vi "process_maxes.vi"(1 "Parsed formula node reference fn 2nd derivative":T1 {"Y Values" format="%.2f"}, 2 "Maxes":dbl[][](array[numeric]), 3 "Wavelengths":dbl[](array[numeric])) -> (0 "Phase''":dbl[](array[numeric]))   [LabVIEW 2022 SP3]
uses:
  <vilib>/gmath/NI_Gmath.lvlib
panel:
  # "operator"
  # "register1"
  # "register2"
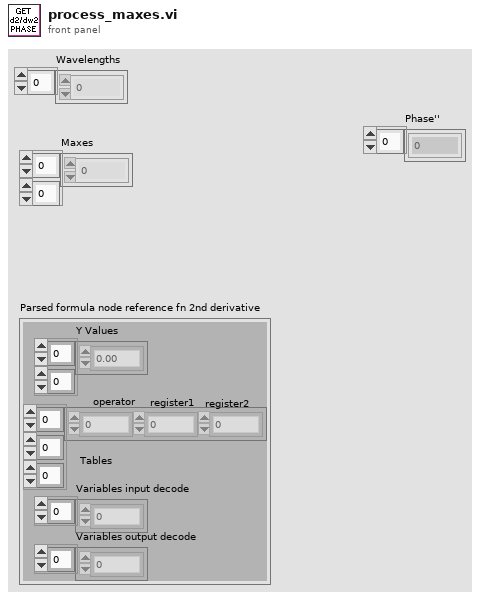
[diagram p1: front panel]
types:
  T1 = cluster{"Y Values":dbl[][], "Tables":i32[][][], "Variables input decode":i32[], "Variables output decode":i32[]}
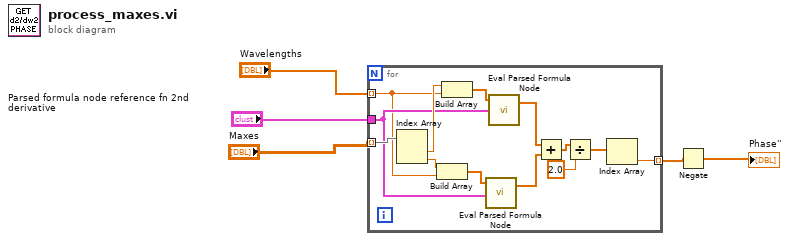
[diagram p0: block diagram]
diagram:
  n1 = for {
    tunnel: "Wavelengths" -> [w13] mode=indexing
    tunnel: "Maxes" -> [w18] mode=indexing
    tunnel: "Parsed formula node reference fn 2nd derivative" -> [w14]
    tunnel: [w7] -> w2 mode=indexing
    n2 = Index Array(array=w18) -> (element #1=w17:dbl, element #2=w6:dbl)  [unwired: 2 in]
    n3 = Build Array(w6, w13) -> (w15:dbl[])
    n4 = Build Array(w17, w13) -> (w16:dbl[])
    n5 = call <vilib>:"Eval Parsed Formula Node.vi"("Parsed Formula Node"=w14, "Input Values"=w15) -> ("Output Values"=w11:dbl[])  [unwired: 1 in, 1 out]
    n6 = call <vilib>:"Eval Parsed Formula Node.vi"("Parsed Formula Node"=w14, "Input Values"=w16) -> ("Output Values"=w12:dbl[])  [unwired: 1 in, 1 out]
    n7 = Add(x=w12, y=w11) -> (x+y=w10:dbl[])
    n8 = Divide(x=w10, y=2.0) -> (x/y=w8:dbl[])
    n9 = Index Array(array=w8) -> (element=w7:dbl)  [unwired: 1 in]
  }
  n10 = Negate(x=w2) -> (-x=→"Phase''":dbl[])
